vi "ConvertModuleTypes.vi"(9 "Module TypeIn":T2 items=["SPC-600"=600, "SPC-630"=630, "SPC-700"=700, "SPC-730"=730, "SPC-130"=130, "SPC-830"=830, "SPC-140"=140, "SPC-930"=930, "DPC-230"=230, "SPC-150"=150, "SPC-150 N"=151, "SPC-150 NX"=152, "SPC-130 EM"=131, "SPC-130 EMN"=132, "SPC-130IN"=135, "SPC-130INX"=136, "SPC-130INXX"=137, "SPC-160"=160, "SPC-160 X"=161, "SPC-160 PCIE"=162, "SPC-180 N"=180, "SPC-180 NX"=181, "SPC-180 NXX"=182, "SPC-180 N-USB"=185, "SPC-180 NX-USB"=186, "SPC-180 NXX-USB"=187, "SPC-QC-104"=104, "SPC-QC-004"=4, "SPC-QC-106"=106, "DPC-330"=330, "PMS-800"=800, "SPC-590"=590, "Simulation"=-1], 10 "ModuleTypeStringIn":string, 11 "BHModuleType":T1 format="x%x" items=["SPC-130"=32, "SPC-600"=33, "SPC-630"=34, "SPC-700"=35, "SPC-730"=36, "SPC-830"=37, "SPC-140"=38, "SPC-930"=39, "SPC-150"=40, "DPC-230"=41, "SPC-130EM"=42, "SPC-160"=43, "SPC-150N"=46, "PMS-800"=51, "SPC-150NX"=128, "SPC-160X"=129, "SPC-160PCIE"=130, "SPC-130EMN"=131, "SPC-180N"=132, "SPC-180NX"=133, "SPC-180NXX"=134, "SPC-180N-USB"=135, "SPC-130IN"=136, "SPC-130INX"=137, "SPC-130INXX"=138, "SPC-QC-104"=139, "Simulation"=-1]) -> (1 "BHModuleType":T1 format="x%x" items=["SPC-130"=32, "SPC-600"=33, "SPC-630"=34, "SPC-700"=35, "SPC-730"=36, "SPC-830"=37, "SPC-140"=38, "SPC-930"=39, "SPC-150"=40, "DPC-230"=41, "SPC-130EM"=42, "SPC-160"=43, "SPC-150N"=46, "PMS-800"=51, "SPC-150NX"=128, "SPC-160X"=129, "SPC-160PCIE"=130, "SPC-130EMN"=131, "SPC-180N"=132, "SPC-180NX"=133, "SPC-180NXX"=134, "SPC-180N-USB"=135, "SPC-130IN"=136, "SPC-130INX"=137, "SPC-130INXX"=138, "SPC-QC-104"=139, "Simulation"=-1], 2 "ModuleTypeString":string, 3 "Module TypeOut":T2=151 items=["SPC-600"=600, "SPC-630"=630, "SPC-700"=700, "SPC-730"=730, "SPC-130"=130, "SPC-830"=830, "SPC-140"=140, "SPC-930"=930, "DPC-230"=230, "SPC-150"=150, "SPC-150 N"=151, "SPC-150 NX"=152, "SPC-130 EM"=131, "SPC-130 EMN"=132, "SPC-130IN"=135, "SPC-130INX"=136, "SPC-130INXX"=137, "SPC-160"=160, "SPC-160 X"=161, "SPC-160 PCIE"=162, "SPC-180 N"=180, "SPC-180 NX"=181, "SPC-180 NXX"=182, "SPC-180 N-USB"=185, "SPC-180 NX-USB"=186, "SPC-180 NXX-USB"=187, "SPC-QC-104"=104, "SPC-QC-004"=4, "SPC-QC-106"=106, "DPC-330"=330, "PMS-800"=800, "SPC-590"=590, "Simulation"=-1])   [LabVIEW 2023]
doc: "The module type can be coded in spcmdll in three different styles. This convenience VI converts each of these styles into the other two.\n\n<b>Warning:</b> Only ever connect one of the input terminals\n\nUse this VI when providing information to an SDT- or SET-file.\n\ninfo@becker-hickl.com"
uses:
  SPC_Wrappers/SPC_Controls/ModuleType.ctl
  SPC_Wrappers/SPC_Controls/BHModuleType.ctl
panel:
  out "Number":i16[](array[numeric])
  out "BH":i16[](array[numeric]) format="%.0x"
  # "Warning: Only ever connect one of the input terminals"
  # "debug info"
  # "from Spc_io.c\nModName spc_mod_name[MAX_SPC_APP]={\n  {M_SPC300, \"SPC-300\"},      {M_SPC330, \"SPC-330\"},      {M_SPC400, \"SPC-400\"},\n  {M_SPC430, \"SPC-430\"},      {M_SPC401, \"SPC-401\"},      {M_SPC431, \"SPC-431\"},\n  {M_SPC402, \"SPC-402\"},      {M_SPC432, \"SPC-432\"},      {M_SPC230, \"SPC-230\"},\n  {M_SPC500, \"SPC-500\"},      {M_SPC530, \"SPC-530\"},      {M_SPC505, \"SPC-505\"},\n  {M_SPC535, \"SPC-535\"},      {M_SPC506, \"SPC-506\"},      {M_SPC536, \"SPC-536\"},\n  {M_SPC600, \"SPC-600\"},      {M_SPC630, \"SPC-630\"},      {M_SPC700, \"SPC-700\"},\n  {M_SPC730, \"SPC-730\"},      {M_SPC130, \"SPC-130\"},      {M_SPC830, \"SPC-830\"},\n  {M_SPC140, \"SPC-140\"},      {M_SPC930, \"SPC-930\"},      {M_SPC150, \"SPC-150\"}, \n  {M_DPC230, \"DPC-230\"},      {M_SPC131, \"SPC-130-EM\"},   {M_SPC160, \"SPC-160\"},\n  {M_DPC330, \"DPC-330\"},      {M_DPC590, \"DPC-590\"},      {M_SPC151, \"SPC-150N\"}, \n  {M_SPC152, \"SPC-150NX\"},    {M_SPC161, \"SPC-160X\"},     {M_SPC162, \"SPC-160PCIE\"},\n  {M_SPC132, \"SPC-130-EMN\"},  {M_SPC180, \"SPC-180N\"},     {M_SPC181, \"SPC-180NX\"},\n  {M_SPC182, \"SPC-180NXX\"},   {M_SPC185, \"SPC-180N-USB\"}, {M_SPC135, \"SPC-130IN\"},\n  {M_SPC136, \"SPC-130INX\"},   {M_SPC137, \"SPC-130INXX\"},  {M_TDC104, \"SPC-QC-104\"}\n  };"
  # "x33 PMS-800 d800"
  # "BHModuleType\nfrom SPC_data_file_structre.h :\nbits 11-4   - BH module type\n                       //      meaning of this field values (hex):\n                       //        0x20 -SPC-130, 0x21 - SPC-600, 0x22 - SPC-630,\n                       //        0x23 -SPC-700, 0x24 - SPC-730, 0x25 - SPC-830,\n                       //        0x26 -SPC-140, 0x27 - SPC-930, 0x28 - SPC-150,\n                       //        0x29 -DPC-230, 0x2a - SPC-130EM, 0x2b -SPC-160,\n                       //        0x2e -SPC-150N, 0x80 - SPC-150NX, 0x81 -SPC-160X,\n                       //        0x82 -SPC-160PCIE, 0x83 -SPC-130EMN, 0x84 -SPC-180N,\n                       //        0x85 -SPC-180NX,   0x86 -SPC-180NXX, 0x87 -SPC-180N-USB,\n                       //        0x88 -SPC-130IN,   0x89 -SPC-130INX, 0x8a -SPC-130INXX\n                       //        0x8b -TDC-104"
  # "Module Type\nfrom Spcm_def.h :\n#define M_WRONG_TYPE  -1\n#define M_SPC600    600   /* PCI version of 400 + 401 + 402 */  \n#define M_SPC630    630   /* PCI version of 430 + 431 + 432 */  \n#define M_SPC700    700   /* PCI version of 500 + 505 + 506 */  \n#define M_SPC730    730   /* PCI version of 530 + 535 + 536 */  \n#define M_SPC130    130   \n#define M_SPC830    830   \n#define M_SPC140    140   \n#define M_SPC930    930   \n#define M_DPC230    230   \n#define M_SPC150    150   \n#define M_SPC151    151    // SPC-150N = SPC-150 with faster discriminators and reduced timing wobble\n#define M_SPC152    152    // SPC-150NX = SPC-150N with changed TAC range ( instead of 50-5000ns):\n                           //       2 variants: SPC-150NX 25-2500ns and \n                           //                   SPC-150NXX (old SPC-150NX-12) 12.5-125ns\n#define M_SPC131    131    // SPC-130-EM  = SPC130 with extended memory ( also known as SPC131 )\n#define M_SPC132    132    // SPC-130-EMN = SPC130 with extended memory, \n                           //      faster discriminators and reduced timing wobble ( also known as SPC132 )\n#define M_SPC135    135    // SPC-130IN - as SPC-130-EMN but with faster data transfer on PCI-EX bus \n                           //                          (using SmartLogic IP_CORE on Xilinx Artix 7)\n#define M_SPC136    136    // SPC-130INX = SPC-130IN with TAC range 25-2500ns ( instead of 50-5000ns)\n#define M_SPC137    137    // SPC-130INXX = SPC-130IN with TAC range 12.5-125ns ( instead of 50-5000ns)\n\n#define M_SPC160    160    // SPC-160 - Special module for optical tomography\n#define M_SPC161    161    // SPC-160X = SPC-160 with TAC range 25-2500ns ( instead of 50-5000ns)\n#define M_SPC162    162    // SPC-160PCIE = SPC-160 on PCI-EX bus\n#define M_SPC180    180    // SPC-180N - as SPC-160  but with faster data transfer on PCI-EX bus \n                           //                           (using SmartLogic IP_CORE on Xilinx Artix 7)\n#define M_SPC181    181    // SPC-180NX = SPC-180N with TAC range 25-2500ns ( instead of 50-5000ns)\n#define M_SPC182    182    // SPC-180NXX = SPC-180N with TAC range 12.5-125ns ( instead of 50-5000ns)\n#define M_SPC185    185    // SPC-180N-USB - as SPC-180N with USB-3 interface \n#define M_SPC186    186    // SPC-180NX-USB - as SPC-180N-USB with TAC range 25-2500ns (instead of 50-5000ns)\n#define M_SPC187    187    // SPC-180NXX-USB - as SPC-180N-USB with TAC range 12.5-125ns (instead of 50-5000ns)\n\n#define M_TDC104    104    // SPC-QC-104  - four channels module ( named TDC-104 further )\n\n#define M_DPC330    330    // DPC330 - Special version of DPC230\n#define M_DPC590    590    // DPC590 - Special version of DPC230"
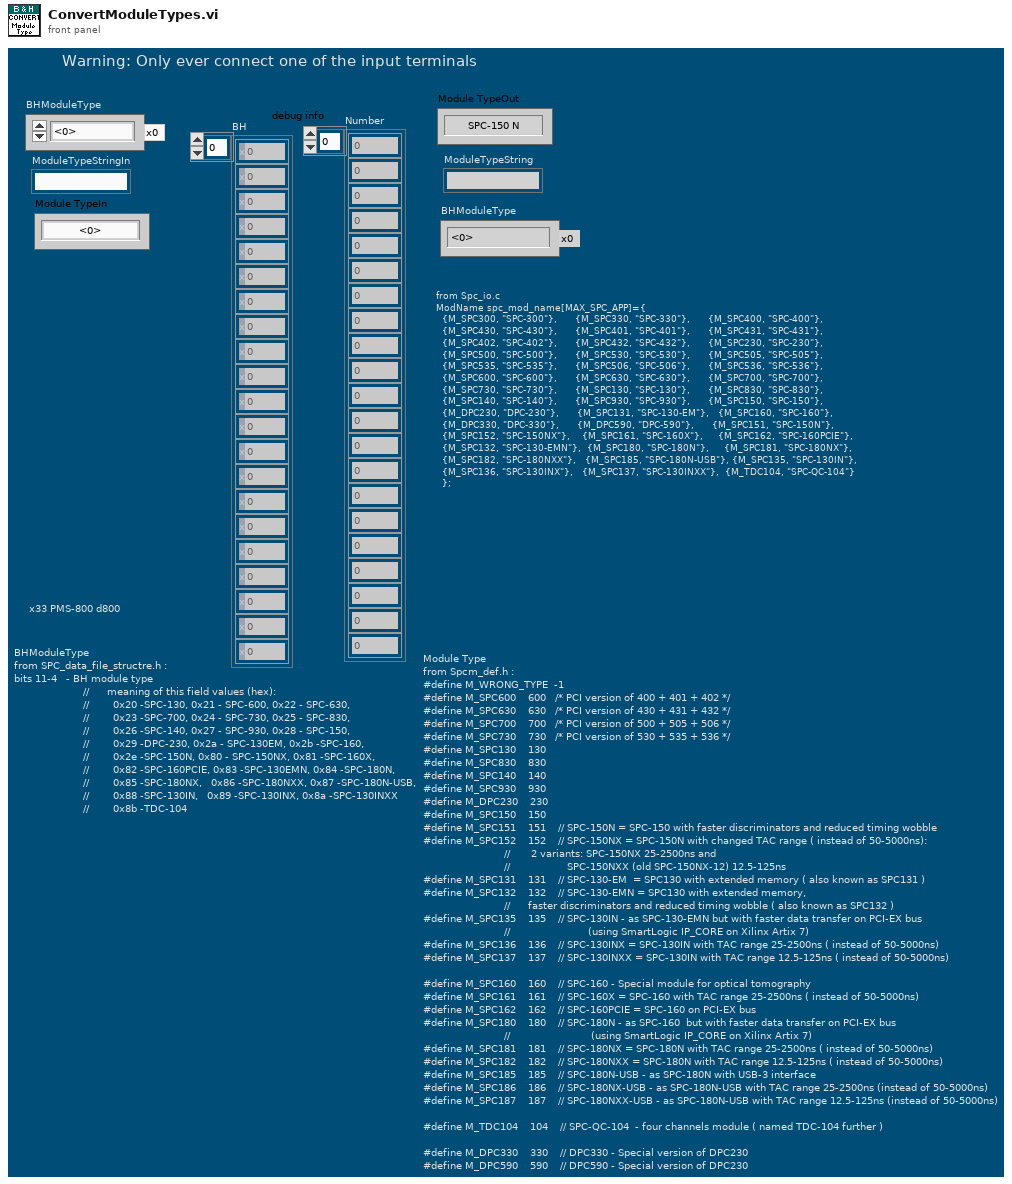
[diagram p1: front panel]
types:
  T1 = typedef "BHModuleType.ctl" = i16
  T2 = typedef "ModuleType.ctl" = i16
  T3 = typedef "LVStringsAndValuesArrayTypeDef_I16.ctl" = cluster{"String":string, "Value":i16}[]
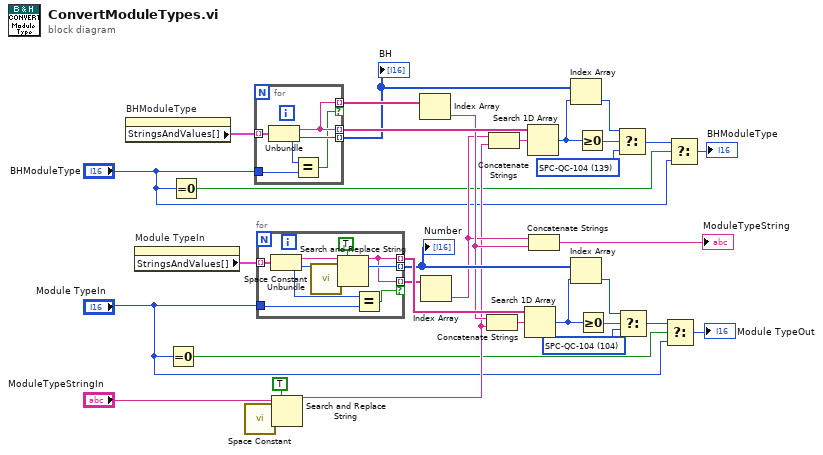
[diagram p0: block diagram]
diagram:
  w9 = T1 139 items=["SPC-130"=32, "SPC-600"=33, "SPC-630"=34, "SPC-700"=35, "SPC-730"=36, "SPC-830"=37, "SPC-140"=38, "SPC-930"=39, "SPC-150"=40, "DPC-230"=41, "SPC-130EM"=42, "SPC-160"=43, "SPC-150N"=46, "SPC-150NX"=128, "SPC-160X"=129, "SPC-160PCIE"=130, "SPC-130EMN"=131, "SPC-180N"=132, "SPC-180NX"=133, "SPC-180NXX"=134, "SPC-180N-USB"=135, "SPC-130IN"=136, "SPC-130INX"=137, "SPC-130INXX"=138, "SPC-QC-104"=139, "Simulation"=-1] ("BHModuleType")
  w10 = T2 104 items=["SPC-600"=600, "SPC-630"=630, "SPC-700"=700, "SPC-730"=730, "SPC-130"=130, "SPC-830"=830, "SPC-140"=140, "SPC-930"=930, "DPC-230"=230, "SPC-150"=150, "SPC-150 N"=151, "SPC-150 NX"=152, "SPC-130 EM"=131, "SPC-130 EMN"=132, "SPC-160"=160, "SPC-160 X"=161, "SPC-160 PCIE"=162, "SPC-180 N"=180, "SPC-180 NX"=181, "SPC-180 NXX"=182, "SPC-180 N-USB"=185, "SPC-180 NX-USB"=186, "SPC-180 NXX-USB"=187, "SPC-QC-104"=104, "DPC-330"=330, "SPC-590"=590, "Simulation"=-1] ("Module TypeIn")
  n1 = property on="BHModuleType" class="Ring (strict)"() -> ("StringsAndValues[]"=w25:T3)  [unwired: 2 in, 2 out]
  n2 = property on="Module TypeIn" class="Ring (strict)"() -> ("StringsAndValues[]"=w33:T3)  [unwired: 2 in, 2 out]
  n3 = Equal To 0?(x="Module TypeIn") -> (x = 0?=w2:bool)
  n4 = Equal To 0?(x="BHModuleType") -> (x = 0?=w8:bool)
  n5 = call <vilib>:"Space Constant.vi"() -> ("String"=w23:string)
  n6 = for {
    tunnel: w25 -> [w38] mode=indexing
    tunnel: "BHModuleType" -> [w37]
    tunnel: [w35] -> w32 mode=indexing
    tunnel: [w36] -> w17 mode=indexing
    tunnel: [w35] -> w30 mode=indexing if=w34
    n7 = Unbundle(w38) -> ("String"=w35:string, "Value"=w36:i16)
    n8 = Equal?(x=w36, y=w37) -> (x = y?=w34:bool)
  }
  "BH" <- w17
  n9 = for {
    tunnel: w33 -> [w46] mode=indexing
    tunnel: "Module TypeIn" -> [w45]
    tunnel: [w39] -> w31 mode=indexing
    tunnel: [w44] -> w28 mode=indexing
    tunnel: [w39] -> w29 mode=indexing if=w43
    n10 = Unbundle(w46) -> ("String"=w40:string, "Value"=w44:i16)
    n11 = call <vilib>:"Space Constant.vi"() -> ("String"=w42:string)
    n12 = Search and Replace String(replace all?=TRUE ("replace all? (F)"), input string=w40, search string=w42) -> (result string=w39:string)  [unwired: 5 in, 3 out]
    n13 = Equal?(x=w44, y=w45) -> (x = y?=w43:bool)
  }
  "Number" <- w28
  n14 = Search and Replace String(replace all?=TRUE ("replace all? (F)"), input string="ModuleTypeStringIn", search string=w23) -> (result string=w18:string)  [unwired: 5 in, 3 out]
  n15 = Index Array(array=w30) -> (element=w27:string)  [unwired: 1 in]
  n16 = Index Array(array=w29) -> (element=w20:string)  [unwired: 1 in]
  n17 = Concatenate Strings(w27, w18) -> (w21:string)
  n18 = Concatenate Strings(w20, w18) -> (w19:string)
  n19 = Search 1D Array(1D array=w31, element=w21) -> (index of element=w16:i32)  [unwired: 1 in]
  n20 = Search 1D Array(1D array=w32, element=w19) -> (index of element=w12:i32)  [unwired: 1 in]
  n21 = Concatenate Strings(w20, w27) -> (→"ModuleTypeString":string)
  n22 = Index Array(array=w17, index=w12) -> (element=w11:i16)
  n23 = Index Array(array=w28, index=w16) -> (element=w14:i16)
  n24 = Greater Or Equal To 0?(x=w12) -> (x >= 0?=w13:bool)
  n25 = Greater Or Equal To 0?(x=w16) -> (x >= 0?=w15:bool)
  n26 = Select(t=w11, s=w13, f=w9) -> (s? t:f=w7:T1)
  n27 = Select(t=w14, s=w15, f=w10) -> (s? t:f=w4:T2)
  n28 = Select(t=w4, s=w2, f="Module TypeIn") -> (s? t:f=→"Module TypeOut":T2)
  n29 = Select(t=w7, s=w8, f="BHModuleType") -> (s? t:f=→"BHModuleType":T1)
